vi "Process File.vi"(8 "error in (no error)":errorcluster, 10 "File":refnum<class "Acquired Result.lvclass">, 11 "NHMFL Synthesizer in":refnum<class "NHMFL Synthesizer.lvclass">) -> (0 "error out":errorcluster, 2 "File out":refnum<class "Acquired Result.lvclass">, 3 "NHMFL Synthesizer out":refnum<class "NHMFL Synthesizer.lvclass">)   [LabVIEW 2018, in "NHMFL Synthesizer.lvclass"]
uses:
  NHMFL Synthesizer.lvclass
  NHMFL_Core/Libraries/Instruments/Results/Acquired Result/Acquired Result.lvclass
  NHMFL Synthesizer.lvclass/NHMFL Synthesizer.ctl
  Read NHMFL Synthesizer Configuration.vi
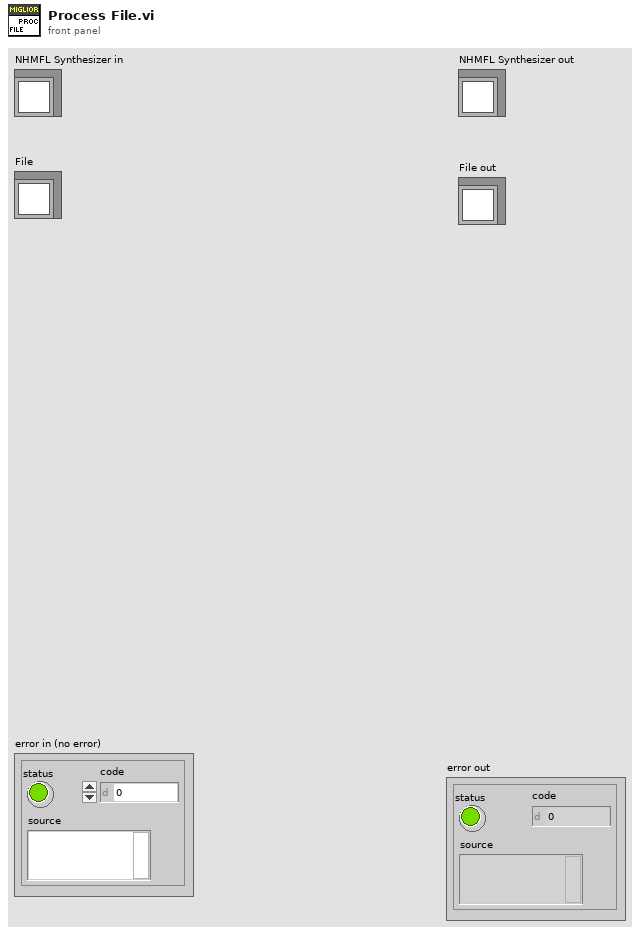
[diagram p1: front panel]
types:
  T1 = enum16{"open", "open or create", "create or replace", "create", "open (read-only)"}
  T2 = typedef "NHMFL Synthesizer Configuration.ctl" = cluster{"DAQmx Device":tag, "Variable amplitude frequency":dbl, "Fixed amplitude frequency":dbl, "Amplitude":dbl, "Clock multiplier":i32, "Channel names (variable F)":string[], "Channel names (fixed F)":string[], "Group":string, "Auto-update other modules":bool, "Recorder module":string, "Lock-in module ":string}
  T3 = typedef "Lockin Parameters.ctl" = cluster{"Frequency":dbl, "Phase":dbl, "Syncronous":bool, "Points per sine wave":i32, "DDS":bool, "Frequency word":u32, "Phase word":u32, "DDS modulus":i64, "DDS clock":dbl}
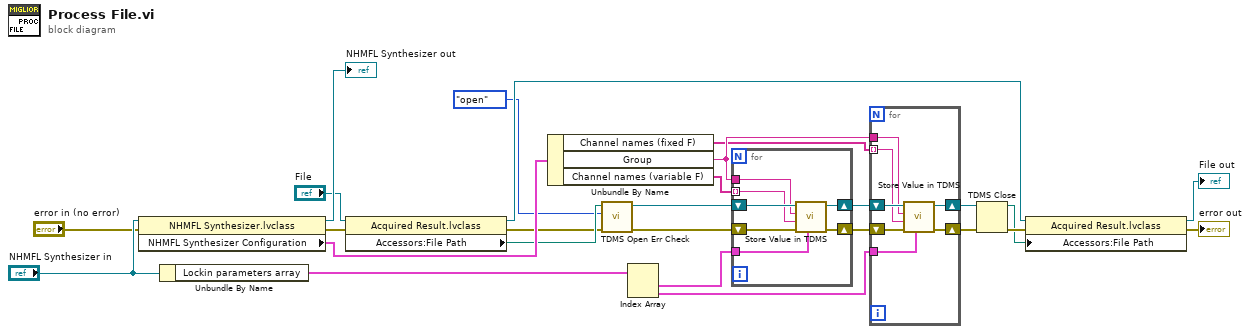
[diagram p0: block diagram]
diagram:
  n1 = property class="NHMFL Synthesizer.lvclass"(reference="NHMFL Synthesizer in", error in="error in (no error)") -> (reference out=→"NHMFL Synthesizer out":refnum<class "NHMFL Synthesizer.lvclass">, error out=w11:errorcluster, "NHMFL Synthesizer Configuration"=w23:T2)
  n2 = Unbundle By Name("NHMFL Synthesizer in") -> ("Lockin parameters array"=w21:T3[])
  n3 = property class="Acquired Result.lvclass"(reference="File", error in=w11) -> (reference out=w6:refnum<class "Acquired Result.lvclass">, error out=w4:errorcluster, "Accessors:File Path"=w5:path)
  n4 = Unbundle By Name(w23) -> ("Channel names (fixed F)"=w13:string[], "Group"=w18:string, "Channel names (variable F)"=w22:string[])
  n5 = call "TDMS Open Err Check.vi"("Error In"=w4, "operation (0:open)"=T1."open", "File Path Control"=w5) -> ("Error Out"=w3:errorcluster, "tdms file out"=w2:refnum<k34>)  [unwired: 6 in, 1 out]
  n6 = Index Array(array=w21) -> (element #1=w20:T3, element #2=w19:T3)  [unwired: 2 in]
  n7 = for {
    tunnel: w22 -> [w29] mode=indexing
    shift-right: [w32] -> w16
    shift-left: w2 -> [w33]
    shift-right: [w31] -> w17
    shift-left: w3 -> [w28]
    tunnel: w18 -> [w30]
    tunnel: w20 -> [w27]
    n8 = call "Store Value in TDMS.vi"("Value"=w27, "Error In"=w28, "channel name"=w29, "group name"=w30, "tdms file"=w33) -> ("Error Out"=w31:errorcluster, "tdms file out"=w32:refnum<k34>)  [unwired: 3 in, 2 out]
  }
  n9 = for {
    tunnel: w13 -> [w36] mode=indexing
    shift-right: [w39] -> w15
    shift-left: w16 -> [w40]
    shift-right: [w38] -> w14
    shift-left: w17 -> [w35]
    tunnel: w18 -> [w37]
    tunnel: w19 -> [w34]
    n10 = call "Store Value in TDMS.vi"("Value"=w34, "Error In"=w35, "channel name"=w36, "group name"=w37, "tdms file"=w40) -> ("Error Out"=w38:errorcluster, "tdms file out"=w39:refnum<k34>)  [unwired: 3 in, 2 out]
  }
  n11 = TDMS Close(8:w14, 11:w15) -> (0:w10:errorcluster, 3:w7:path)
  n12 = property class="Acquired Result.lvclass"(reference=w6, error in=w10, "Accessors:File Path"=w7) -> (reference out=→"File out":refnum<class "Acquired Result.lvclass">, error out=→"error out":errorcluster)
